vi "RT Check to Activate.vi"() -> ()   [LabVIEW 2022 SP3]
panel:
  in  "y":dbl format="%#_13g"
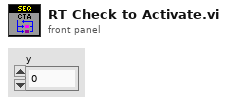
[diagram p1: front panel]
types:
  T1 = cluster{"CDT":dbl, "Range":dbl, "Component ID":string}[]
  T2 = cluster{"CDT":dbl, "Position":bool, "Component ID":string}[]
  T3 = cluster{"CDT":dbl, "Position":bool, "Component ID":string}
  T4 = cluster{"CDT":dbl, "Range":dbl, "Component ID":string}
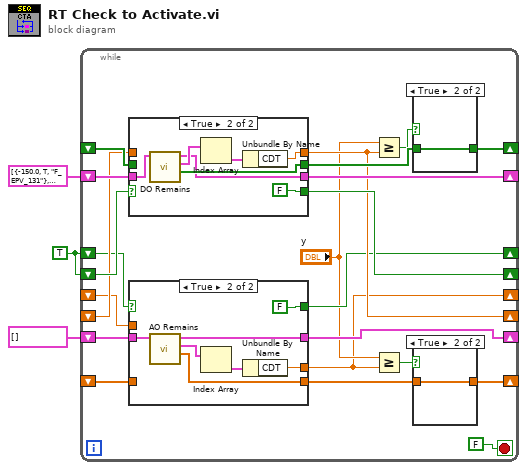
[diagram p0: block diagram]
diagram:
  w2 = TRUE
  n1 = while {
    shift-right: [w24] -> _
    shift-left: T2 [{"CDT"=-150.0, "Position"=TRUE, "Component ID"="F_EPV_131"}, {"CDT"=-150.0, "Position"=TRUE, "Component ID"="F_EPV_131"}, {"CDT"=-135.0, "Position"=FALSE, "Component ID"="F_EPV_132"}, {"CDT"=-120.0, "Position"=FALSE, "Component ID"="F_EPV_131"}, {"CDT"=-20.0, "Position"=TRUE, "Component ID"="F_EPV_136"}, {"CDT"=-10.0, "Position"=FALSE, "Component ID"="F_EPV_136"}] ("DO") -> [w25]
    shift-right: [w17] -> _
    shift-left: w2 -> [w23]
    shift-right: [w4] -> _
    shift-left: _ -> [w21]
    shift-right: [w16] -> _
    shift-left: _ -> [w20]
    shift-right: [w9] -> _
    shift-left: _ -> [w15]
    shift-right: [w14] -> _
    shift-left: T1 [] ("Remains AO") -> [w13]
    shift-right: [w12] -> _
    shift-left: w2 -> [w7]
    shift-right: [w6] -> _
    shift-left: _ -> [w5]
    stop <- FALSE stop-if-true
    n2 = case shown="True" w23 {
      selector: w23 -> [w41 _]
      tunnel: w25 -> [w42 w51]
      tunnel: [w42 w46] -> w24
      tunnel: [w44 w48] -> w19
      tunnel: w21 -> [w44 _]
      tunnel: [w43 w47] -> w16
      tunnel: w20 -> [w43 _]
      tunnel: [w41 FALSE] -> w17
      frame False {
      }
      frame True {
        n3 = call "DO Remains.vi"("Array"=w51) -> ("DO value"=w48:bool[], "Same DO"=w50:T2, "Remains"=w46:T2)  [unwired: 8 in]
        n4 = Index Array(array=w50) -> (element=w49:T3)  [unwired: 1 in]
        n5 = Unbundle By Name(w49) -> ("CDT"=w47:dbl)
      }
    }
    n6 = case shown="True" w7 {
      selector: w7 -> [w29 _]
      tunnel: w13 -> [w30 w38]
      tunnel: [w30 w34] -> w14
      tunnel: [w31 w35] -> w9
      tunnel: w15 -> [w31 _]
      tunnel: [w29 FALSE] -> w12
      tunnel: [w28 w32] -> w8
      tunnel: w5 -> [w28 _]
      frame False {
      }
      frame True {
        n7 = call "AO Remains.vi"("Array"=w38) -> ("AO"=w32:dbl[], "Same AO"=w37:T1, "Remains AO"=w34:T1)  [unwired: 8 in]
        n8 = Index Array(array=w37) -> (element=w36:T4)  [unwired: 1 in]
        n9 = Unbundle By Name(w36) -> ("CDT"=w35:dbl)
      }
    }
    n10 = Greater Or Equal?(x="y", y=w16) -> (x >= y?=w18:bool)
    n11 = Greater Or Equal?(x="y", y=w9) -> (x >= y?=w11:bool)
    n12 = case shown="True" w18 {
      tunnel: w19 -> [w39 w40]
      tunnel: [w39 w40] -> w4
      frame False {
      }
      frame True {
      }
    }
    n13 = case shown="True" w11 {
      tunnel: w8 -> [w26 w27]
      tunnel: [w26 w27] -> w6
      frame False {
      }
      frame True {
      }
    }
  }
